vi "Data Analog aquired.vi"(8 "error in":errorcluster, 10 "data":waveform(dbl)[](array[waveform])) -> (0 "error out":errorcluster)   [LabVIEW 2020, in "Acquisition.lvlib"]
doc: "se recibio la info de analog\n_____\nCreated using Delacor QMH Event Scripter 6.0.0.121."
uses:
  Acquisition.lvlib
  Data Analog aquired Argument--cluster.ctl
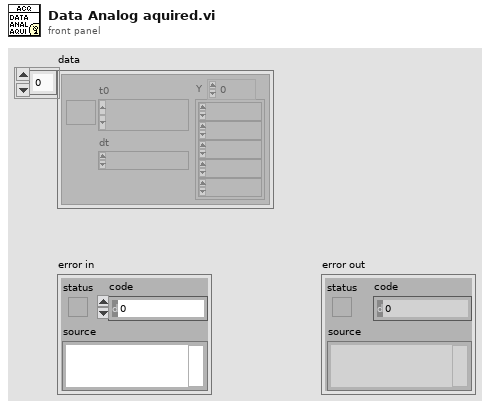
[diagram p1: front panel]
types:
  T1 = typedef "Acquisition.lvlib/Data Analog aquired Argument--cluster.ctl" = cluster{"data":waveform(dbl)[]}
  T2 = typedef "Acquisition.lvlib/Broadcast Events--cluster.ctl" = cluster{"Module Did Init":refnum<user-event>, "Status Updated":refnum<user-event>, "Error Reported":refnum<user-event>, "Module Did Stop":refnum<user-event>, "Update Module Execution Status":refnum<user-event>, "Data Analog aquired":refnum<user-event>, "DIGITAL DATA":refnum<user-event>, "TIPO ADQUI":refnum<user-event>}
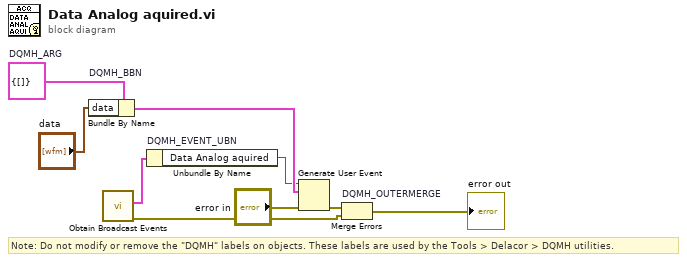
[diagram p0: block diagram]
diagram:
  w4 = T1 {"data"=[]}  # DQMH_ARG
  # "Note: Do not modify or remove the \"DQMH\" labels on objects. These labels are used by the Tools > Delacor > DQMH utilities."
  n1 = Bundle By Name "DQMH_BBN"(cluster=w4, "data"="data") -> (w7:T1)
  n2 = call "Obtain Broadcast Events.vi"() -> ("error out"=w2:errorcluster, "Acquisition Broadcast Events"=w1:T2)  [unwired: 10 in]
  n3 = Unbundle By Name "DQMH_EVENT_UBN"(w1) -> ("Data Analog aquired"=w6:refnum<user-event>)
  n4 = Generate User Event(user event=w6, event data cluster=w7, error in="error in") -> (error out=w5:errorcluster)  [unwired: 1 in, 1 out]
  n5 = Merge Errors "DQMH_OUTERMERGE"(w5, w2) -> (→"error out":errorcluster)
